vi "test_Find FPGA Addon.vi"(8 "error in (no error)":errorcluster, 11 "TestCase in":refnum<class "FPGA Addon Scripting API Unit Tests.lvclass">) -> (0 "error out":errorcluster, 3 "TestCase out":refnum<class "FPGA Addon Scripting API Unit Tests.lvclass">)   [LabVIEW 2020, in "FPGA Addon Scripting API Unit Tests.lvclass"]
uses:
  FPGA Addon Scripting API Unit Tests.lvclass
  <vilib>/addons/_JKI Toolkits/VI Tester/TestCase.llb/TestCase.lvclass
  FPGA Addon Test Class/FPGA Addon Test Class.lvclass
  <vilib>/NI VeriStand/Custom Device Tools/Custom Device Utility Library/Custom Device Utility Library.lvlib
  APIs/Scripting API/Scripting API.lvlib
  C:/Program Files (x86)/National Instruments/LabVIEW 2020/vi.lib/addons/_JKI Toolkits/VI Tester/TestCase.llb/TestCase.lvclass
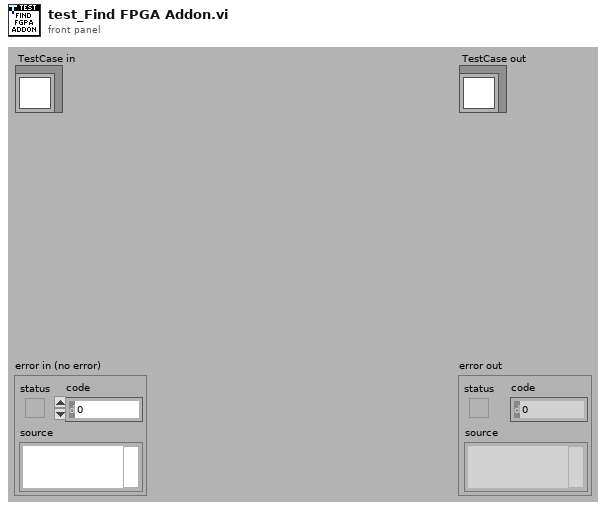
[diagram p1: front panel]
types:
  T1 = typedef "Custom Device API.lvlib/Custom Device Item Ref.ctl" = u64
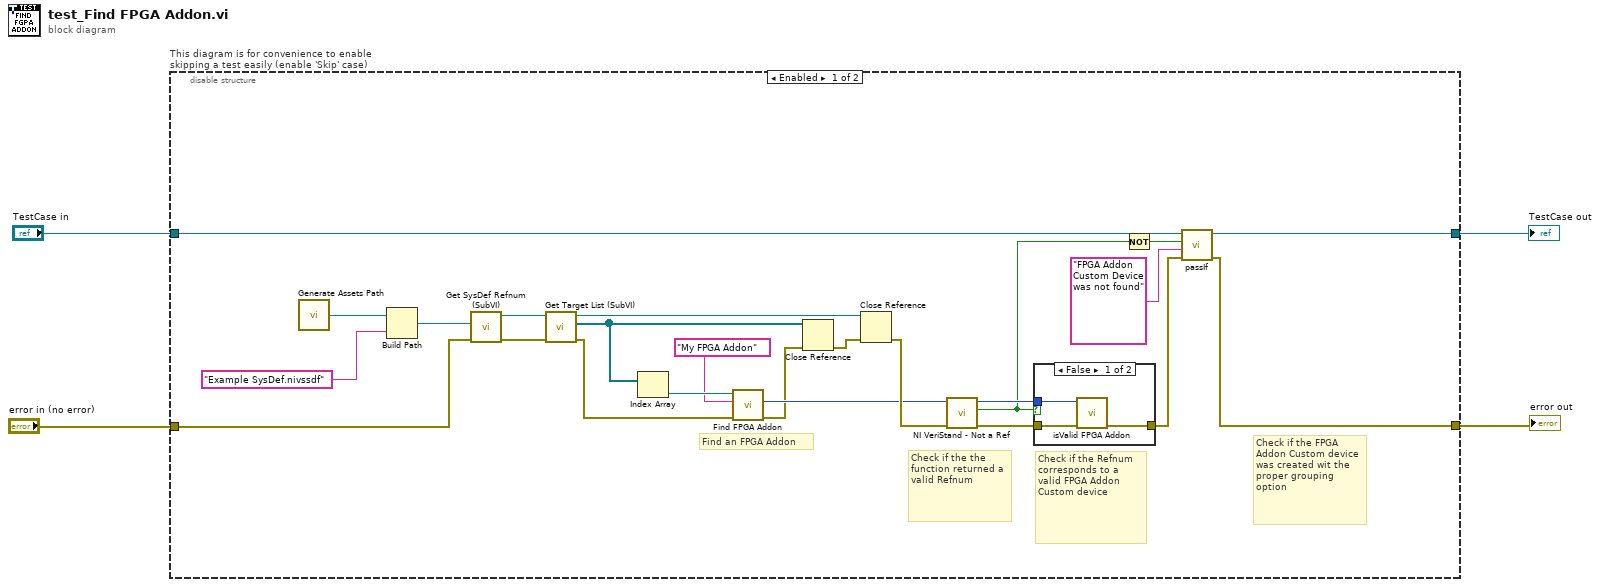
[diagram p0: block diagram]
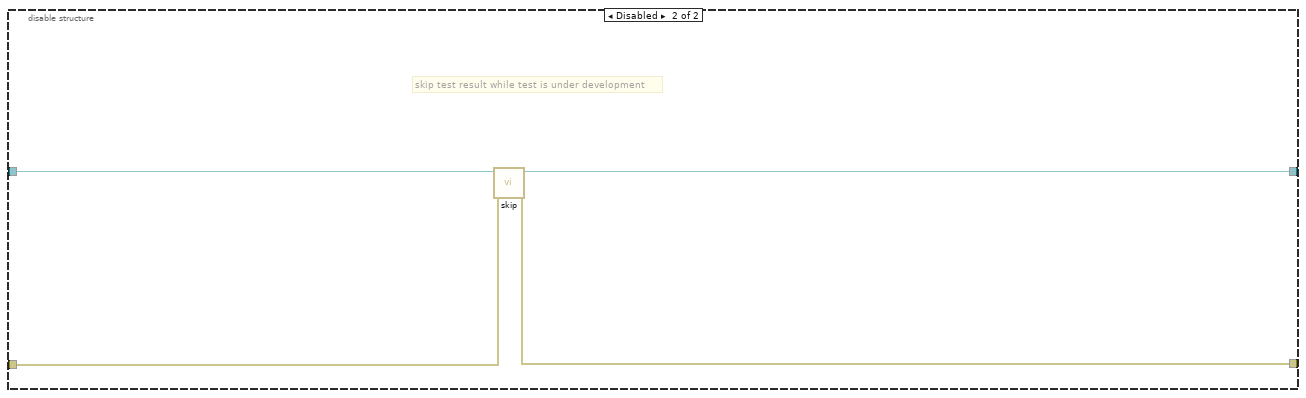
[diagram p3: hidden frame]
diagram:
  n1 = disable-structure "This diagram is for convenience to enable skipping a test easily (enable 'Skip' case)" shown="Enabled" {
    disable-tunnel: "TestCase in" -> [w22 w36]
    disable-tunnel: [w7 w34] -> w1
    disable-tunnel: [w6 w35] -> w3
    disable-tunnel: "error in (no error)" -> [w24 w33]
    frame Enabled {
      # "Check if the FPGA Addon Custom device was created wit the proper grouping option"
      # "Check if the Refnum corresponds to a valid FPGA Addon Custom device"
      # "Check if the the function returned a valid Refnum"
      # "Find an FPGA Addon"
      n2 = call "Generate Assets Path.vi"() -> ("Assets path"=w28:path)
      n3 = Build Path(base path=w28, name or relative path="Example SysDef.nivssdf") -> (appended path=w26:path)
      n4 = call "Get SysDef Refnum (SubVI).vi"("error in (no error)"=w24, "System Definition path"=w26) -> ("error out"=w23:errorcluster, "SysDef Refnum out"=w25:refnum<k24>)  [unwired: 8 in]
      n5 = call "Get Target List (SubVI).vi"("error in (no error)"=w23, "SysDef Refnum in"=w25) -> ("error out"=w11:errorcluster, "Target List Refnums"=w19:refnum<k24>[], "SysDef Refnum out"=w18:refnum<k24>)  [unwired: 7 in]
      n6 = Index Array(array=w19) -> (element=w12:refnum<k24>)  [unwired: 1 in]
      n7 = call "Find FPGA Addon.vi"("error in"=w11, "FPGA addon name"="My FPGA Addon", "target in"=w12) -> ("error out"=w8:errorcluster, "FPGA addon refnum out"=w9:T1)  [unwired: 5 in, 2 out]
      n8 = Close Reference(reference=w19, error in (no error)=w8) -> (error out=w17:errorcluster)
      n9 = Close Reference(reference=w18, error in (no error)=w17) -> (error out=w16:errorcluster)
      n10 = call <vilib>:"NI VeriStand - Not a Ref.vi"("error in (no error)"=w16, "Item Ref"=w9) -> ("error out"=w14:errorcluster, "Not a Ref"=w5:bool, "Item Ref out"=w15:T1)  [unwired: 7 in]
      n11 = case shown="False" w5 {
        tunnel: w15 -> [w31 _]
        tunnel: w14 -> [w30 w32]
        tunnel: [w29 w32] -> w13
        frame False {
          n12 = call "isValid FPGA Addon.vi"("error in"=w30, "FPGA Addon refnum in"=w31) -> ("error out"=w29:errorcluster)  [unwired: 8 in, 1 out]
        }
        frame True {
        }
      }
      n13 = Not(x=w5) -> (.not. x?=w21:bool)
      n14 = call-dynamic "passIf.vi"("error in (no error)"=w13, "message (\"\")"="FPGA Addon Custom Device was not found" ("message (\"\")"), "pass"=w21, "TestCase in"=w22) -> ("error out"=w6:errorcluster, "TestCase out"=w7:refnum<class "FPGA Addon Scripting API Unit Tests.lvclass">)  [unwired: 6 in]
    }
    frame Disabled {
      # "skip test result while test is under development"
      n15 = call <vilib>:"skip.vi"("error in (no error)"=w33, "TestCase in"=w36) -> ("error out"=w35:errorcluster, "TestCase out"=w34:refnum<class "FPGA Addon Scripting API Unit Tests.lvclass">)  [unwired: 8 in]
    }
  }
  "error out" <- w3
  "TestCase out" <- w1
